vi "PingCore.vi"(8 "error in (no error)":errorcluster, 11 "MicronTemplateAPIs in":refnum<class "MicronTemplateAPIs.lvclass">) -> (0 "error out":errorcluster, 2 "Response":string, 3 "MicronTemplateAPIs out":refnum<class "MicronTemplateAPIs.lvclass">)   [LabVIEW 2019, in "MicronTemplateAPIs.lvlib" / "MicronTemplateAPIs.lvclass"]
uses:
  MicronTemplateAPIs.lvclass
  gRPC/Client/MicronGRPCClient.lvclass
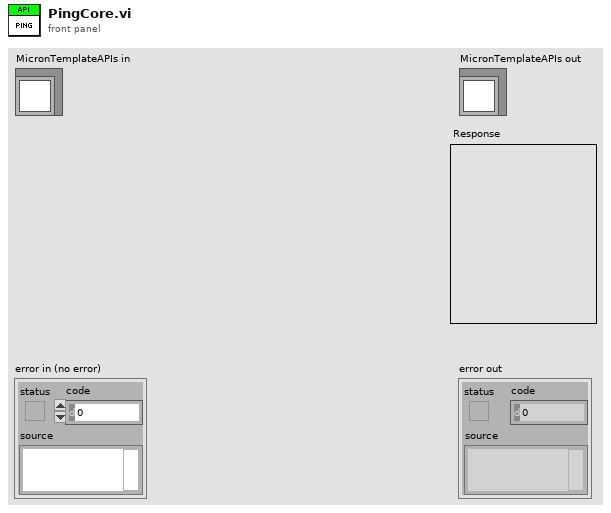
[diagram p1: front panel]
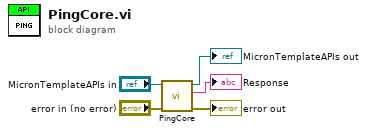
[diagram p0: block diagram]
diagram:
  n1 = call-parent "PingCore.vi"("error in (no error)"="error in (no error)", "MicronClient in"="MicronTemplateAPIs in") -> ("error out"=→"error out":errorcluster, "Response"=→"Response":string, "MicronClient out"=→"MicronTemplateAPIs out":refnum<class "MicronTemplateAPIs.lvclass">)  [unwired: 7 in]
